vi "Set IConfiguration.vi"(8 "error in":errorcluster, 10 "IConfiguration":refnum<class "IConfiguration.lvclass">, 11 "IHasConfiguration in":refnum<class "IHas Configuration.lvclass">) -> (0 "error out":errorcluster, 3 "IHasConfiguration out":refnum<class "IHas Configuration.lvclass">)   [LabVIEW 2019, in "IHas Configuration.lvclass"]
uses:
  IHas Configuration.lvclass
  IConfiguration/IConfiguration.lvclass
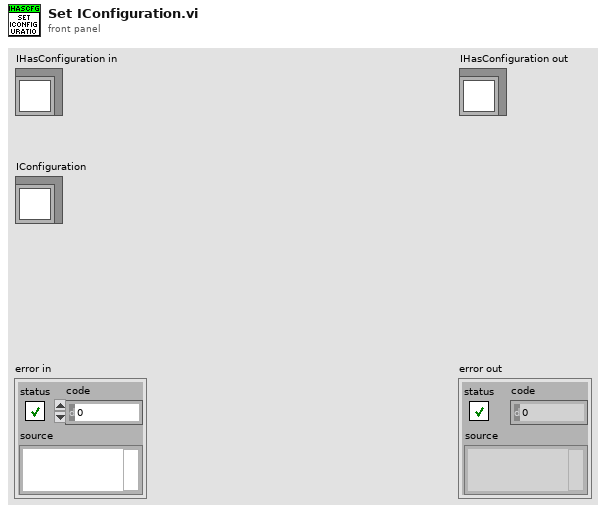
[diagram p1: front panel]
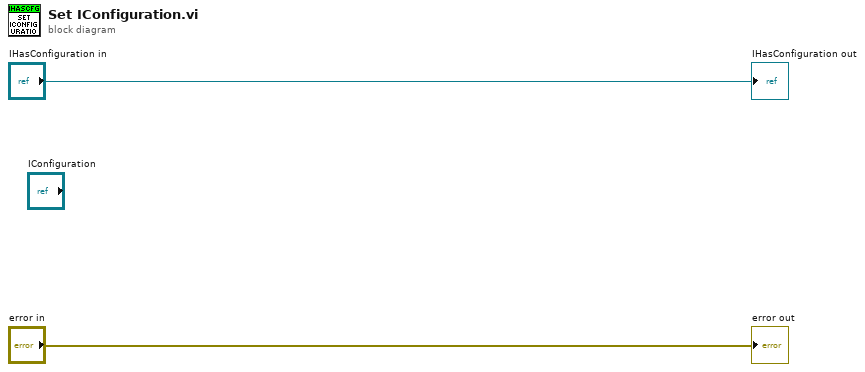
[diagram p0: block diagram]
diagram:
  "error out" <- "error in"
  "IHasConfiguration out" <- "IHasConfiguration in"
